vi "Exit Variable.vi"() -> ()   [LabVIEW 2021]
panel:
  out "Global Variable Exit":bool
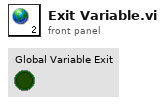
[diagram p1: front panel]
diagram:
